vi "AE_data_read_final.vi"() -> ()   [LabVIEW 2009]
panel:
  in  "Number of data points saved":i32=1000
  in  "Time window (ms)":i32=50
  out "Sum of data points arrived within time window":dbl
  out "Time running (ms)":i32
  out "Array of last values":dbl[][](array[numeric])
  out "Last value received from data socket":dbl
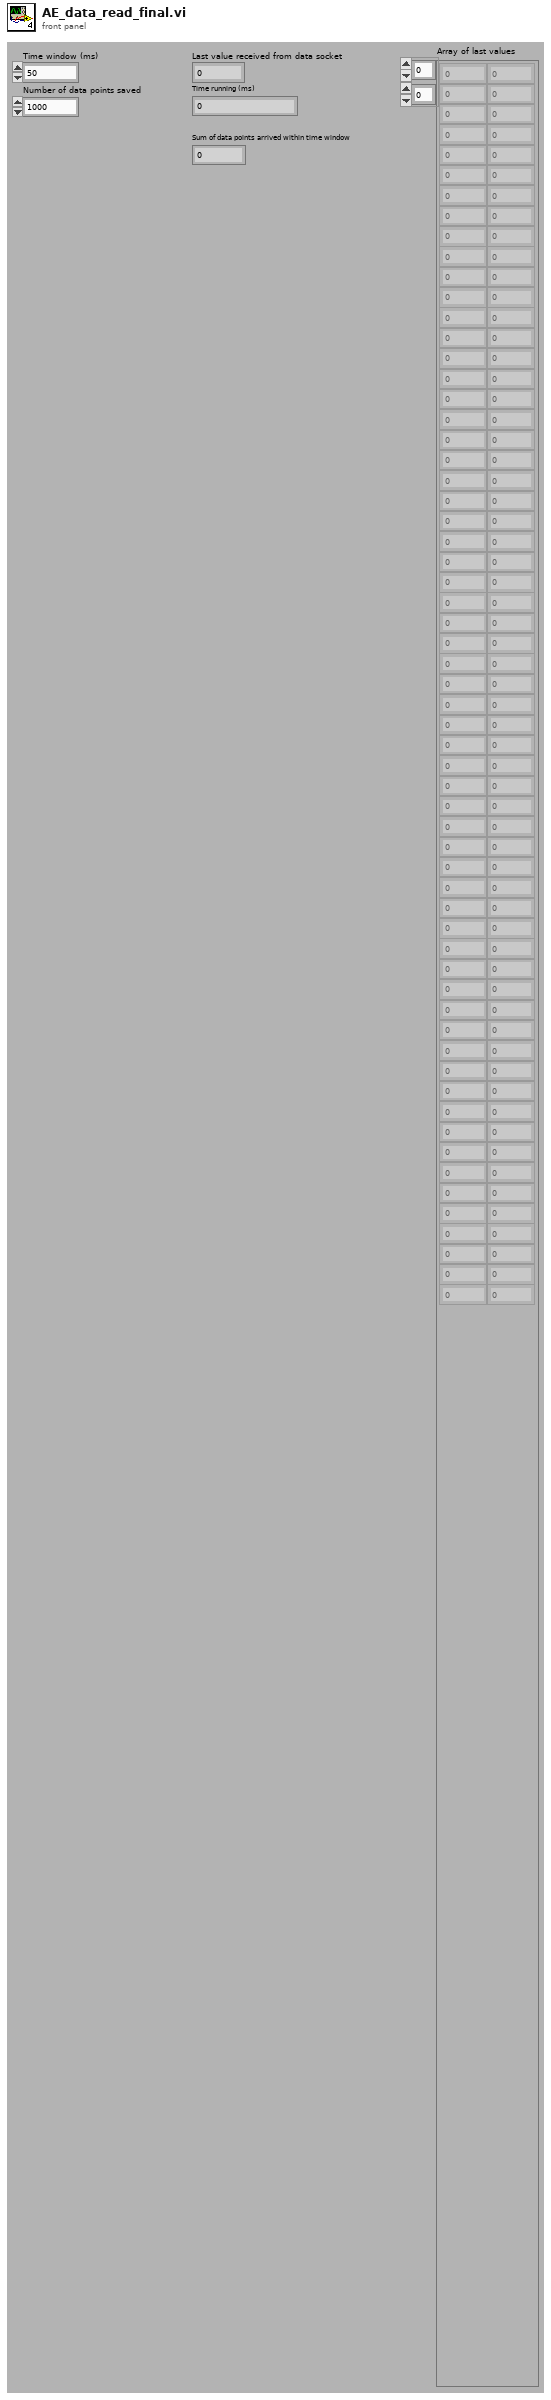
[diagram p1: front panel]
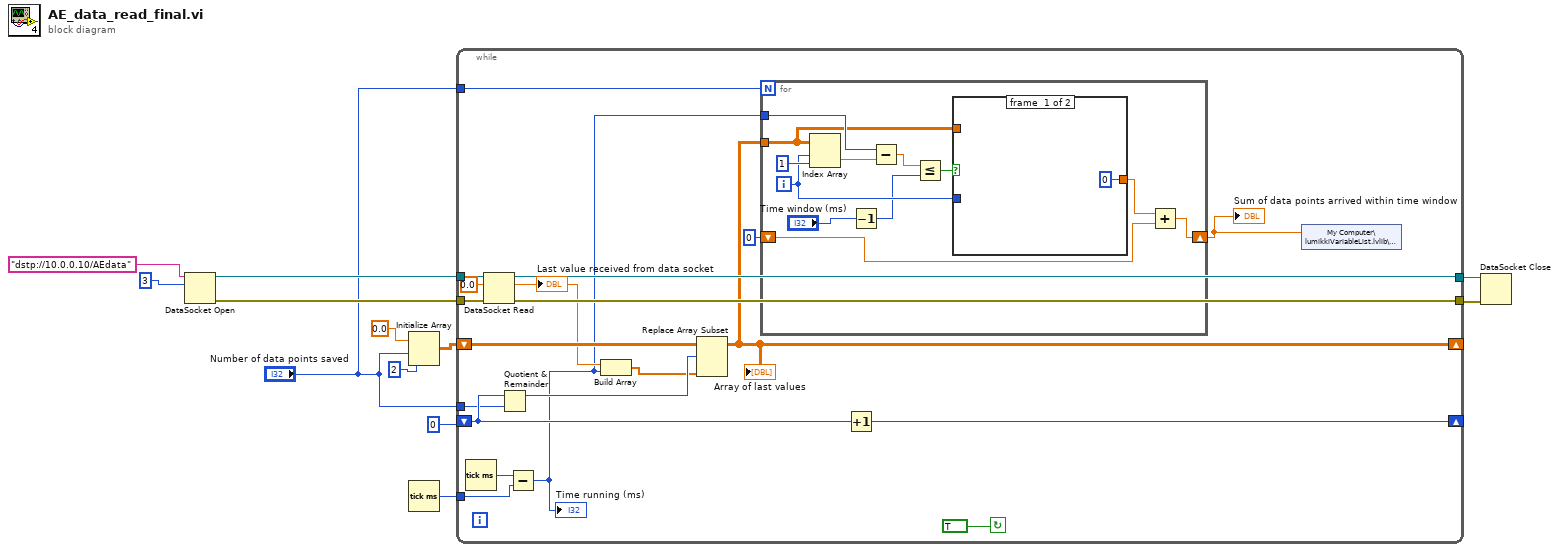
[diagram p0: block diagram]
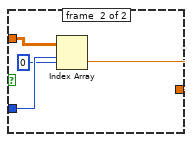
[diagram p2: hidden frame]
diagram:
  n1 = DataSocket Open(10:3, 11:"dstp://10.0.0.10/AEdata") -> (0:w9:errorcluster, 3:w10:refnum<k13>)  [unwired: 1 in, 1 out]
  n2 = Initialize Array(0.0, "Number of data points saved", 2) -> (w5:dbl[][])
  n3 = Tick Count (ms)() -> (millisecond timer value=w6:u32)
  n4 = while {
    tunnel: w10 -> [w32]
    tunnel: w9 -> [w31]
    tunnel: [w29] -> w8
    tunnel: [w28] -> w7
    tunnel: w6 -> [w25]
    shift-right: [w15] -> _
    shift-left: w5 -> [w24]
    shift-right: [w23] -> _
    shift-left: 0 -> [w22]
    tunnel: "Number of data points saved" -> [w21]
    tunnel: "Number of data points saved" -> [w18]
    stop <- TRUE continue-if-true
    n5 = Tick Count (ms)() -> (millisecond timer value=w27:u32)
    n6 = DataSocket Read(8:w31, 10:0.0, 11:w32) -> (0:w28:errorcluster, 2:w19:dbl, 3:w29:refnum<k13>)  [unwired: 6 out]
    "Last value received from data socket" <- w19
    n7 = Quotient & Remainder(x=w22, y=w21) -> (x-y*floor(x/y)=w20:i32)  [unwired: 1 out]
    n8 = Subtract(x=w27, y=w25) -> (x-y=w17:u32)
    "Time running (ms)" <- w17
    n9 = Build Array(w19, w17) -> (w16:dbl[])
    n10 = Replace Array Subset(array=w24, new element=w16, index (row)=w20) -> (w15:dbl[][])  [unwired: 1 in]
    "Array of last values" <- w15
    n11 = for {
      N: w18 -> [_]
      tunnel: w17 -> [w43]
      tunnel: w15 -> [w39]
      shift-right: [w35] -> w13
      shift-left: 0 -> [w36]
      i -> [w38]
      n12 = Index Array(array=w39, index (row)=w38, index (col)=1) -> (element=w42:dbl)
      n13 = Decrement(x="Time window (ms)") -> (x-1=w34:i32)
      n14 = Subtract(x=w43, y=w42) -> (x-y=w40:dbl)
      n15 = Less Or Equal?(x=w40, y=w34) -> (x <= y?=w41:bool)
      n16 = case shown="True" w41 {
        tunnel: w39 -> [_ w49]
        tunnel: w38 -> [_ w48]
        tunnel: [0 w46] -> w37
        frame #0 {
        }
        frame #1 {
          n17 = Index Array(array=w49, index (row)=w48, index (col)=0) -> (element=w46:dbl)
        }
      }
      n18 = Add(x=w37, y=w36) -> (x+y=w35:dbl)
    }
    "Sum of data points arrived within time window" <- w13
    n19 = Increment(x=w22) -> (x+1=w23:i32)
    n20 = shared-variable "My Computer\\lumikkiVariableList.lvlib\\AEdataSum"(w13) -> ()  [unwired: 1 in, 1 out]
  }
  n21 = DataSocket Close(8:w7, 11:w8) -> ()  [unwired: 3 out]
